vi "Scale Controls.vi"(6 "Initialize group (false)":bool, 7 "rules":string, 8 "error in (no error)":errorcluster, 9 "pane size":T3, 10 "Decorations on Pane":refnum<vi>[](array[refnum]), 11 "Controls on Pane":refnum<vi>[](array[refnum])) -> (0 "error out":errorcluster)   [LabVIEW 2020]
doc: "Simple and schmutzig VI that will scale controls and labeled decorations by delta change of pane size.\nUsage: put in multiline string with rules:\nmy control name a [edge:LRTB]\nmy control name b [edge:LRB]\n...\n\nwhere edge:LRTB defines edges to be sticked to pane. LR - scale horizontaly, R - no scale, move object only, TB - scale vertically, B - just stick object to bottom, no scaling...\nWhen using for decorations, name them first with script 'Set Decoration Label'!"
uses:
  <vilib>/Utility/miscctls.llb/LVRectTypeDef.ctl
  Scale Controls List.ctl
  Scale Controls Record.ctl
  <vilib>/regexp/Match Regular Expression.xnode
panel:
  in  "lists":T1[](array[typedef])
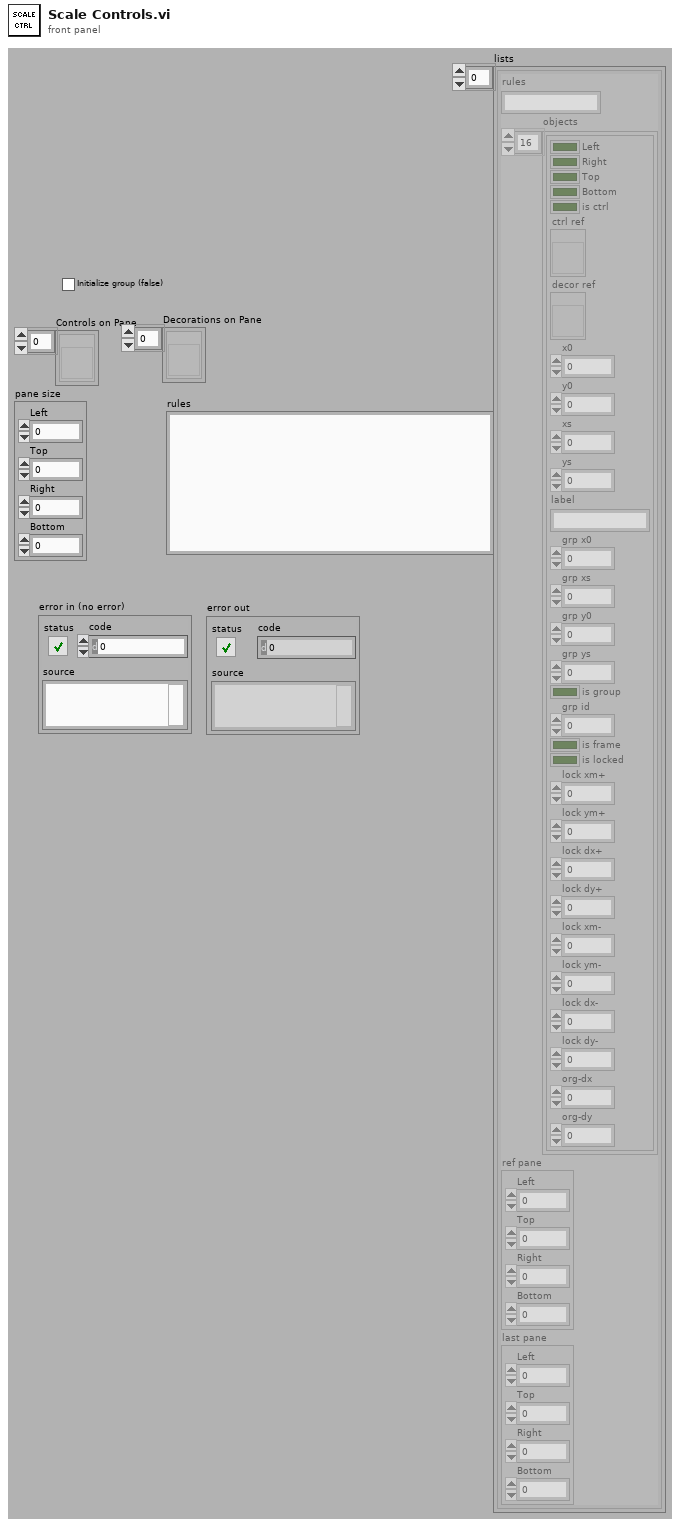
[diagram p1: front panel]
types:
  T1 = typedef "Scale Controls List.ctl" = cluster{"rules":string, "objects":T2[], "ref pane":T3, "last pane":T3}
  T2 = typedef "Scale Controls Record.ctl" = cluster{"Left":bool, "Right":bool, "Top":bool, "Bottom":bool, "is ctrl":bool, "ctrl ref":refnum<vi>, "decor ref":refnum<vi>, "x0":i32, "y0":i32, "xs":i32, "ys":i32, "label":string, "grp x0":i32, "grp xs":i32, "grp y0":i32, "grp ys":i32, "is group":bool, "grp id":i32, "is frame":bool, "is locked":bool, "lock xm+":i32, "lock ym+":i32, "lock dx+":i32, "lock dy+":i32, "lock xm-":i32, "lock ym-":i32, "lock dx-":i32, "lock dy-":i32, "org-dx":i32, "org-dy":i32}
  T3 = typedef "LVRectTypeDef.ctl" = cluster{"Left":i16, "Top":i16, "Right":i16, "Bottom":i16}
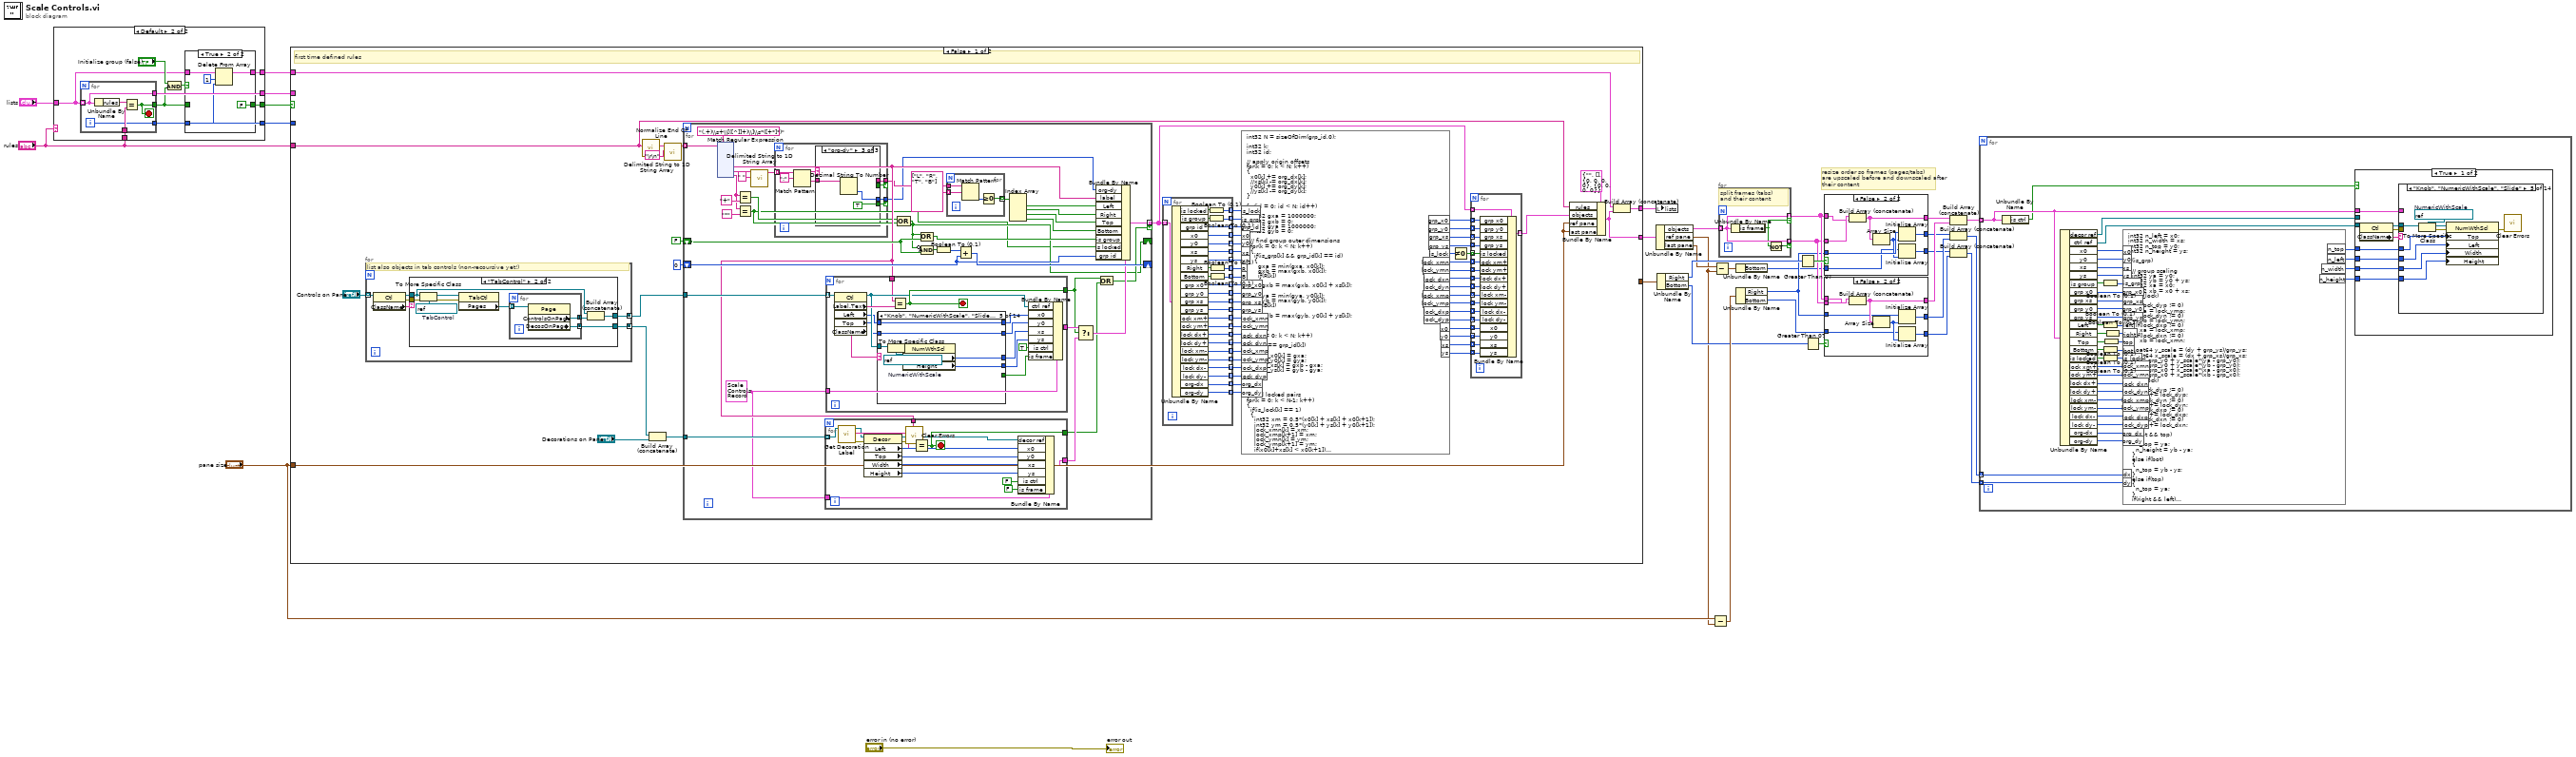
[diagram p0: block diagram]
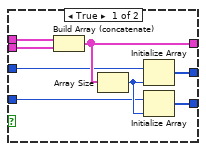
[diagram p2: hidden frame]
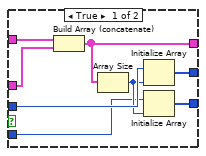
[diagram p3: hidden frame]
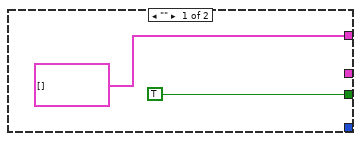
[diagram p4: hidden frame]
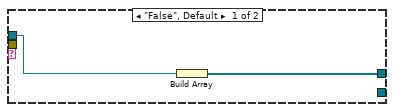
[diagram p6: hidden frame]
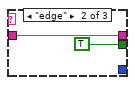
[diagram p8: hidden frame]
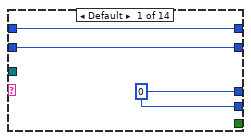
[diagram p9: hidden frame]
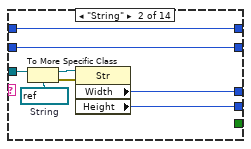
[diagram p10: hidden frame]
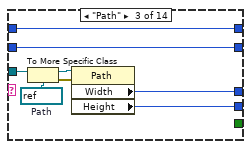
[diagram p11: hidden frame]
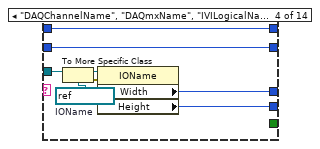
[diagram p12: hidden frame]
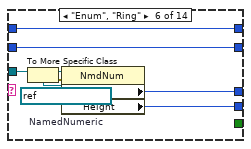
[diagram p13: hidden frame]
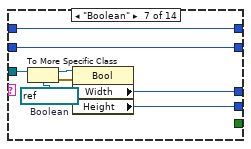
[diagram p14: hidden frame]
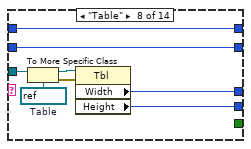
[diagram p15: hidden frame]
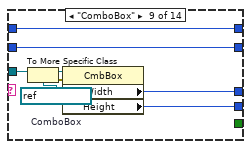
[diagram p16: hidden frame]
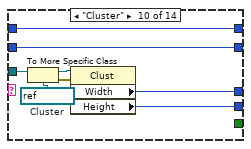
[diagram p17: hidden frame]
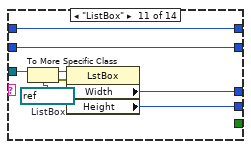
[diagram p18: hidden frame]
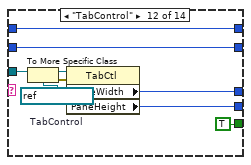
[diagram p19: hidden frame]
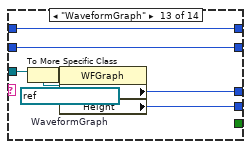
[diagram p20: hidden frame]
diagram:
  # "resize order so frames (pages/tabs)\nare upscaled before and downscaled after\ntheir content"
  n1 = case shown="Default" "rules" {
    tunnel: [TRUE w40] -> w33
    tunnel: [_ w45] -> w31
    tunnel: "rules" -> [_ w44]
    tunnel: [T1[] [] ("lists") w38] -> w29
    tunnel: "lists" -> [_ w39]
    tunnel: [_ w37] -> w9
    frame "" {
    }
    frame Default {
      n2 = for {
        tunnel: w39 -> [w54] mode=indexing
        tunnel: w44 -> [w56]
        tunnel: [w55] -> w41
        tunnel: [w54] -> w45
        tunnel: [w53] -> w37
        i -> [w53]
        stop <- w55 stop-if-true
        n3 = Unbundle By Name(w54) -> ("rules"=w57:string)
        n4 = Equal?(x=w57, y=w56) -> (x = y?=w55:bool)
      }
      n5 = Compound Arithmetic op=AND("Initialize group (false)", w41) -> (w42:bool)
      n6 = case shown="True" w42 {
        tunnel: [w47 FALSE] -> w40
        tunnel: w41 -> [w47 _]
        tunnel: w39 -> [w46 w52]
        tunnel: [w46 w51] -> w38
        tunnel: w37 -> [_ w49]
        frame False {
        }
        frame True {
          n7 = Delete From Array(array=w52, length=1, index=w49) -> (array with subset deleted=w51:T1[])  [unwired: 1 out]
        }
      }
    }
  }
  n8 = case shown="False" w33 {
    tunnel: "rules" -> [w112 _]
    tunnel: w29 -> [w111 w500]
    tunnel: [w110 w499] -> w32
    tunnel: [w109 w498] -> w30
    tunnel: w31 -> [_ w502]
    tunnel: "pane size" -> [w88 w495]
    tunnel: w9 -> [_ w497]
    tunnel: [_ w501] -> w8
    frame False {
      # "first time defined rules"
      n9 = for {
        tunnel: "Controls on Pane" -> [w122] mode=indexing
        tunnel: [w118] -> w61 mode=concatenating
        tunnel: [w117] -> w60 mode=concatenating
        # "list also objects in tab controls (non-recoursive yet!)"
        n10 = property class="Ctl"(reference=w122) -> (reference out=w119:refnum<vi>, error out=w120:errorcluster, "ClassName"=w121:string)  [unwired: 1 in]
        n11 = case shown="\"TabControl\"" w121 {
          tunnel: w120 -> [_ w130]
          tunnel: w119 -> [w124 w127]
          tunnel: [w123 w126] -> w118
          tunnel: [_ w125] -> w117
          frame "False", Default {
            n12 = Build Array(w124) -> (w123:refnum<vi>[])
          }
          frame "TabControl" {
            w131 = refnum<vi> refnum  # TabControl
            n13 = To More Specific Class(target class=w131, reference=w127, error in=w130) -> (specific class reference=w133:refnum<vi>, error out=w132:errorcluster)
            n14 = property class="TabCtl"(reference=w133, error in=w132) -> ("Pages"=w129:refnum<vi>[])  [unwired: 2 out]
            n15 = for {
              tunnel: w129 -> [w136] mode=indexing
              tunnel: [w135] -> w128 mode=concatenating
              tunnel: [w134] -> w125 mode=concatenating
              n16 = property class="Page"(reference=w136) -> ("ControlsOnPage"=w135:refnum<vi>[], "DecosOnPage"=w134:refnum<vi>[])  [unwired: 1 in, 2 out]
            }
            n17 = Build Array (concatenate)(w127, w128) -> (w126:refnum<vi>[])
          }
        }
      }
      n18 = call <vilib>:"Normalize End Of Line.vi"("string in"=w112) -> ("string out"=w114:string)  [unwired: 7 in]
      n19 = Build Array (concatenate)(w60, "Decorations on Pane") -> (w58:refnum<vi>[])
      n20 = call <vilib>:"Delimited String to 1D String Array.vi"("delimiter"="\r\n", "delimited string"=w114) -> ("string array"=w115:string[])  [unwired: 9 in]
      n21 = for {
        tunnel: w115 -> [w219] mode=indexing
        tunnel: [w210] -> w95 mode=indexing if=w195
        tunnel: w61 -> [w211]
        shift-right: [w191] -> _
        shift-left: FALSE -> [w208]
        shift-right: [w205] -> _
        shift-left: 0 -> [w204]
        tunnel: w58 -> [w203]
        w201 = T2 {"Left"=FALSE, "Right"=FALSE, "Top"=FALSE, "Bottom"=FALSE, "is ctrl"=FALSE, "ctrl ref"=refnum, "decor ref"=refnum, "x0"=0, "y0"=0, "xs"=0, "ys"=0, "label"="", "grp x0"=0, "grp xs"=0, "grp y0"=0, "grp ys"=0, "is group"=FALSE, "grp id"=0, "is frame"=FALSE, "is locked"=FALSE, "lock xm+"=0, "lock ym+"=0, "lock dx+"=0, "lock dy+"=0, "lock xm-"=0, "lock ym-"=0, "lock dx-"=0, "lock dy-"=0, "org-dx"=0, "org-dy"=0} ("object")
        n22 = xnode "Match Regular Expression"("input string"=w219, "regular expression"="(.+)\\s+\\[([^]]+)\\]\\s*([+*]*)") -> ("submatch 1"=w202:string, "submatch 2"=w188:string, "submatch 3"=w189:string)  [unwired: 4 in, 5 out]
        n23 = Equal?(x=w189, y="+") -> (x = y?=w192:bool)
        n24 = Equal?(x=w189, y="*") -> (x = y?=w190:bool)
        n25 = call <vilib>:"Delimited String to 1D String Array.vi"("delimiter"=" ", "delimited string"=w188) -> ("string array"=w186:string[])  [unwired: 9 in]
        n26 = for {
          tunnel: w186 -> [w227] mode=indexing
          tunnel: [w223] -> w185 if=w222
          tunnel: [w221] -> w184 if=w220
          n27 = Match Pattern(string=w227, regular expression=":") -> (before substring=w225:string, after substring=w224:string)  [unwired: 1 in, 2 out]
          n28 = case shown="\"org-dy\"" w225 {
            tunnel: [_ w229 _] -> w223
            tunnel: w224 -> [_ w229 w232]
            tunnel: [_ TRUE _] -> w222
            tunnel: [_ _ w231] -> w221
            tunnel: [_ _ TRUE] -> w220
            frame Default {
            }
            frame "edge" {
            }
            frame "org-dy" {
              n29 = Decimal String To Number(string=w232) -> (number=w231:i32)  [unwired: 2 in, 1 out]
            }
          }
        }
        n30 = for {
          tunnel: w203 -> [w237] mode=indexing
          tunnel: w202 -> [w244]
          tunnel: w201 -> [w243]
          tunnel: [w246] -> w199
          tunnel: [w245] -> w196
          stop <- w245 stop-if-true
          n31 = call "Get Decoration Label.vi"("Decor Refnum"=w237) -> ("error out"=w238:errorcluster, "Label"=w239:string, "dup Decor Refnum"=w236:refnum<vi>)  [unwired: 4 in]
          n32 = property class="Decor"(reference=w236, error in=w238) -> (reference out=w235:refnum<vi>, error out=w234:errorcluster, "Left"=w248:i32, "Top"=w242:i32, "Width"=w241:u32, "Height"=w240:u32)
          n33 = call <vilib>:"Clear Errors.vi"("error in (no error)"=w234) -> ()  [unwired: 5 in, 2 out]
          n34 = Equal?(x=w244, y=w239) -> (x = y?=w245:bool)
          n35 = Bundle By Name(cluster=w243, "decor ref"=w235, "x0"=w248, "y0"=w242, "xs"=w241, "ys"=w240, "is ctrl"=FALSE, "is frame"=FALSE) -> (w246:T2)
        }
        n36 = for {
          tunnel: w211 -> [w264] mode=indexing
          tunnel: w202 -> [w257]
          tunnel: w201 -> [w255]
          tunnel: [w261] -> w200
          tunnel: [w260] -> w197
          stop <- w260 stop-if-true
          n37 = property class="Ctl"(reference=w264) -> (reference out=w259:refnum<vi>, "Label.Text"=w263:string, "Left"=w252:i32, "Top"=w250:i32, "ClassName"=w258:string)  [unwired: 1 in, 1 out]
          n38 = case shown="\"Knob\", \"NumericWithScale\", \"Slide\"" w258 {
            tunnel: w259 -> [_ w272 w280 w288 w296 w304 w312 w320 w328 w336 w344 w353 w361 w369]
            tunnel: [w267 w271 w279 w287 w295 w303 w311 w319 w327 w335 w343 w352 w360 w368] -> w256
            tunnel: [w267 w270 w278 w286 w294 w302 w310 w318 w326 w334 w342 w351 w359 w366] -> w254
            tunnel: [_ _ _ _ _ _ _ _ _ _ _ TRUE ("is ctrl") _ _] -> w253
            tunnel: [w265 w269 w277 w285 w293 w301 w309 w317 w325 w333 w341 w349 w358 w367] -> w251
            tunnel: w252 -> [w265 w269 w277 w285 w293 w301 w309 w317 w325 w333 w341 w349 w358 w367]
            tunnel: [w266 w268 w276 w284 w292 w300 w308 w316 w324 w332 w340 w348 w357 w365] -> w249
            tunnel: w250 -> [w266 w268 w276 w284 w292 w300 w308 w316 w324 w332 w340 w348 w357 _]
            frame Default {
              w267 = u32 0 ("Width")
            }
            frame "String" {
              w275 = refnum<vi> refnum  # String
              n39 = To More Specific Class(target class=w275, reference=w272) -> (specific class reference=w273:refnum<vi>, error out=w274:errorcluster)  [unwired: 1 in]
              n40 = property class="Str"(reference=w273, error in=w274) -> ("Width"=w271:u32, "Height"=w270:u32)  [unwired: 2 out]
            }
            frame "Path" {
              w283 = refnum<vi> refnum  # Path
              n41 = To More Specific Class(target class=w283, reference=w280) -> (specific class reference=w281:refnum<vi>, error out=w282:errorcluster)  [unwired: 1 in]
              n42 = property class="Path"(reference=w281, error in=w282) -> ("Width"=w279:u32, "Height"=w278:u32)  [unwired: 2 out]
            }
            frame "DAQChannelName", "DAQmxName", "IVILogicalName", "VISAResourceName" {
              w291 = refnum<vi> refnum  # IOName
              n43 = To More Specific Class(target class=w291, reference=w288) -> (specific class reference=w289:refnum<vi>, error out=w290:errorcluster)  [unwired: 1 in]
              n44 = property class="IOName"(reference=w289, error in=w290) -> ("Width"=w287:u32, "Height"=w286:u32)  [unwired: 2 out]
            }
            frame "Knob", "NumericWithScale", "Slide" {
              w299 = refnum<vi> refnum  # NumericWithScale
              n45 = To More Specific Class(target class=w299, reference=w296) -> (specific class reference=w297:refnum<vi>, error out=w298:errorcluster)  [unwired: 1 in]
              n46 = property class="NumWthScl"(reference=w297, error in=w298) -> ("Width"=w295:u32, "Height"=w294:u32)  [unwired: 2 out]
            }
            frame "Enum", "Ring" {
              w307 = refnum<vi> refnum  # NamedNumeric
              n47 = To More Specific Class(target class=w307, reference=w304) -> (specific class reference=w305:refnum<vi>, error out=w306:errorcluster)  [unwired: 1 in]
              n48 = property class="NmdNum"(reference=w305, error in=w306) -> ("Width"=w303:u32, "Height"=w302:u32)  [unwired: 2 out]
            }
            frame "Boolean" {
              w315 = refnum<vi> refnum  # Boolean
              n49 = To More Specific Class(target class=w315, reference=w312) -> (specific class reference=w313:refnum<vi>, error out=w314:errorcluster)  [unwired: 1 in]
              n50 = property class="Bool"(reference=w313, error in=w314) -> ("Width"=w311:u32, "Height"=w310:u32)  [unwired: 2 out]
            }
            frame "Table" {
              w323 = refnum<vi> refnum  # Table
              n51 = To More Specific Class(target class=w323, reference=w320) -> (specific class reference=w321:refnum<vi>, error out=w322:errorcluster)  [unwired: 1 in]
              n52 = property class="Tbl"(reference=w321, error in=w322) -> ("Width"=w319:u32, "Height"=w318:u32)  [unwired: 2 out]
            }
            frame "ComboBox" {
              w331 = refnum<vi> refnum  # ComboBox
              n53 = To More Specific Class(target class=w331, reference=w328) -> (specific class reference=w329:refnum<vi>, error out=w330:errorcluster)  [unwired: 1 in]
              n54 = property class="CmbBox"(reference=w329, error in=w330) -> ("Width"=w327:u32, "Height"=w326:u32)  [unwired: 2 out]
            }
            frame "Cluster" {
              w339 = refnum<vi> refnum  # Cluster
              n55 = To More Specific Class(target class=w339, reference=w336) -> (specific class reference=w337:refnum<vi>, error out=w338:errorcluster)  [unwired: 1 in]
              n56 = property class="Clust"(reference=w337, error in=w338) -> ("Width"=w335:u32, "Height"=w334:u32)  [unwired: 2 out]
            }
            frame "ListBox" {
              w347 = refnum<vi> refnum  # ListBox
              n57 = To More Specific Class(target class=w347, reference=w344) -> (specific class reference=w345:refnum<vi>, error out=w346:errorcluster)  [unwired: 1 in]
              n58 = property class="LstBox"(reference=w345, error in=w346) -> ("Width"=w343:u32, "Height"=w342:u32)  [unwired: 2 out]
            }
            frame "TabControl" {
              w356 = refnum<vi> refnum  # TabControl
              n59 = To More Specific Class(target class=w356, reference=w353) -> (specific class reference=w354:refnum<vi>, error out=w355:errorcluster)  [unwired: 1 in]
              n60 = property class="TabCtl"(reference=w354, error in=w355) -> ("PaneWidth"=w352:u32, "PaneHeight"=w351:u32)  [unwired: 2 out]
            }
            frame "WaveformGraph" {
              w364 = refnum<vi> refnum  # WaveformGraph
              n61 = To More Specific Class(target class=w364, reference=w361) -> (specific class reference=w362:refnum<vi>, error out=w363:errorcluster)  [unwired: 1 in]
              n62 = property class="WFGraph"(reference=w362, error in=w363) -> ("Width"=w360:u32, "Height"=w359:u32)  [unwired: 2 out]
            }
            frame "XYGraph" {
              w372 = refnum<vi> refnum  # XYGraph
              n63 = To More Specific Class(target class=w372, reference=w369) -> (specific class reference=w370:refnum<vi>, error out=w371:errorcluster)  [unwired: 1 in]
              n64 = property class="XYGraph"(reference=w370, error in=w371) -> ("Width"=w368:u32, "Height"=w366:u32, "Top"=w365:i32)  [unwired: 2 out]
            }
          }
          n65 = Equal?(x=w257, y=w263) -> (x = y?=w260:bool)
          n66 = Bundle By Name(cluster=w255, "ctrl ref"=w259, "x0"=w251, "y0"=w249, "xs"=w256, "ys"=w254, "is ctrl"=TRUE, "is frame"=w253) -> (w261:T2)
        }
        n67 = Compound Arithmetic op=OR(w192, w190) -> (w191:bool)
        n68 = Compound Arithmetic op=OR(w191, w208) -> (w193:bool)
        n69 = Compound Arithmetic op=AND(invert w191, w208) -> (w207:bool)
        n70 = Boolean To (0,1)(Boolean=w207) -> (0, 1=w206:i16)
        n71 = for {
          tunnel: w185 -> [w376]
          tunnel: string[] ["L", "R", "T", "B"] -> [w375] mode=indexing
          tunnel: [w373] -> w216 mode=indexing
          n72 = Match Pattern(string=w376, regular expression=w375) -> (offset past match=w374:i32)  [unwired: 1 in, 3 out]
          n73 = Greater Or Equal To 0?(x=w374) -> (x >= 0?=w373:bool)
        }
        n74 = Add(x=w206, y=w204) -> (x+y=w205:i32)
        n75 = Index Array(array=w216) -> (element #1=w215:bool, element #2=w214:bool, element #3=w213:bool, element #4=w212:bool)  [unwired: 4 in]
        n76 = Select(t=w200, s=w197, f=w199) -> (s? t:f=w198:T2)
        n77 = Bundle By Name(cluster=w198, "org-dy"=w184, "label"=w202, "Left"=w215, "Right"=w214, "Top"=w213, "Bottom"=w212, "is group"=w193, "is locked"=w190, "grp id"=w204) -> (w210:T2)
        n78 = Compound Arithmetic op=OR(w197, w196) -> (w195:bool)
      }
      n79 = for {
        tunnel: w95 -> [w183] mode=indexing
        tunnel: [w181] -> w106 mode=indexing
        tunnel: [w180] -> w89 mode=indexing
        tunnel: [w179] -> w105 mode=indexing
        tunnel: [w178] -> w104 mode=indexing
        tunnel: [w177] -> w103 mode=indexing
        tunnel: [w176] -> w102 mode=indexing
        tunnel: [w174] -> w101 mode=indexing
        tunnel: [w172] -> w100 mode=indexing
        tunnel: [w171] -> w99 mode=indexing
        tunnel: [w170] -> w98 mode=indexing
        tunnel: [w169] -> w97 mode=indexing
        tunnel: [w168] -> w96 mode=indexing
        tunnel: [w166] -> w87 mode=indexing
        tunnel: [w165] -> w80 mode=indexing
        tunnel: [w164] -> w79 mode=indexing
        tunnel: [w163] -> w78 mode=indexing
        tunnel: [w162] -> w77 mode=indexing
        tunnel: [w161] -> w76 mode=indexing
        tunnel: [w160] -> w75 mode=indexing
        tunnel: [w159] -> w74 mode=indexing
        tunnel: [w158] -> w73 mode=indexing
        tunnel: [w157] -> w68 mode=indexing
        tunnel: [w156] -> w67 mode=indexing
        n80 = Unbundle By Name(w183) -> ("is locked"=w167:bool, "is group"=w182:bool, "grp id"=w181:i32, "x0"=w179:i32, "y0"=w178:i32, "xs"=w177:i32, "ys"=w176:i32, "Right"=w175:bool, "Bottom"=w173:bool, "grp x0"=w171:i32, "grp y0"=w170:i32, "grp xs"=w169:i32, "grp ys"=w168:i32, "lock xm+"=w165:i32, "lock ym+"=w164:i32, "lock dx+"=w163:i32, "lock dy+"=w162:i32, "lock xm-"=w161:i32, "lock ym-"=w160:i32, "lock dx-"=w159:i32, "lock dy-"=w158:i32, "org-dx"=w157:i32, "org-dy"=w156:i32)
        n81 = Boolean To (0,1)(Boolean=w167) -> (0, 1=w166:i16)
        n82 = Boolean To (0,1)(Boolean=w182) -> (0, 1=w180:i16)
        n83 = Boolean To (0,1)(Boolean=w175) -> (0, 1=w174:i16)
        n84 = Boolean To (0,1)(Boolean=w173) -> (0, 1=w172:i16)
      }
      n85 = formula code="int32 N = sizeOfDim(grp_id,0);\n\nint32 k;\nint32 id;\n\n// apply origin offsets\nfor(k = 0; k < N; k++)\n{\n  x0[k] += org_dx[k];\n  //xs[k] -= org_dx[k];\n  y0[k] += org_dy[k];\n  //ys[k] -= org_dy[k];\n}\n\nfor(id = 0; id < N; id++)\n{\n  int32 gxa = 1000000;\n  int32 gxb = 0;\n  int32 gya = 1000000;\n  int32 gyb = 0;\n\n  // find group outer dimensions\n  for(k = 0; k < N; k++)\n  {\n    if(is_grp[k] && grp_id[k] == id)\n    {\n      gxa = min(gxa, x0[k]);\n      gxb = max(gxb, x0[k]);\n      if(R[k])\n      {\n        gxb = max(gxb, x0[k] + xs[k]);\n      }\n      gya = min(gya, y0[k]);\n      gyb = max(gyb, y0[k]);\n      if(B[k])\n      {\n        gyb = max(gyb, y0[k] + ys[k]);\n      }\n    }\n  }\n  for(k = 0; k < N; k++)\n  {\n    if(id == grp_id[k])\n    {\n      grp_x0[k] = gxa;\n      grp_y0[k] = gya;\n      grp_xs[k] = gxb - gxa;\n      grp_ys[k] = gyb - gya;\n    }\n  }\n}\n\n// find locked pairs\nfor(k = 0; k < N-1; k++)\n{\n  if(is_lock[k] == 1)\n  {\n    int32 xm = 0.5*(x0[k] + xs[k] + x0[k+1]);\n    int32 ym = 0.5*(y0[k] + ys[k] + y0[k+1]);\n    lock_xmn[k] = xm;\n    lock_xmp[k+1] = xm;\n    lock_ymn[k] = ym;\n    lock_ymp[k+1] = ym;\n    if(x0[k]+xs[k] < x0[k+1])\n    {\n      lock_dxn[k] = (x0[k] + xs[k]) - xm;\n      lock_dxp[k+1] = (x0[k+1]) - xm;\n    }\n    else\n    {\n      lock_dxn[k] = 0;\n      lock_dxp[k+1] = 0;\n    }\n    if(y0[k]+ys[k] < y0[k+1])\n    {\n      lock_dyn[k] = (y0[k] + ys[k]) - ym;\n      lock_dyp[k+1] = (y0[k+1]) - ym;\n    }\n    else\n    {\n      lock_dyn[k] = 0;\n      lock_dyp[k+1] = 0;\n    }\n    if(!is_lock[k+1])\n      is_lock[k+1] = 2;\n  }\n}"("is_grp"=w89, "grp_id"=w106, "x0"=w105, "y0"=w104, "xs"=w103, "ys"=w102, "R"=w101, "B"=w100, "grp_x0"=w99, "grp_y0"=w98, "grp_xs"=w97, "grp_ys"=w96, "is_lock"=w87, "lock_xmn"=w80, "lock_ymn"=w79, "lock_dxn"=w78, "lock_dyn"=w77, "lock_xmp"=w76, "lock_ymp"=w75, "lock_dxp"=w74, "lock_dyp"=w73, "org_dx"=w68, "org_dy"=w67) -> ("grp_x0"=w94:i32[], "grp_y0"=w93:i32[], "grp_xs"=w92:i32[], "grp_ys"=w91:i32[], "is_lock"=w86:i16[], "lock_xmn"=w84:i32[], "lock_ymn"=w83:i32[], "lock_dxn"=w82:i32[], "lock_dyn"=w81:i32[], "lock_xmp"=w72:i32[], "lock_ymp"=w71:i32[], "lock_dxp"=w70:i32[], "lock_dyp"=w69:i32[], "x0"=w66:i32[], "y0"=w65:i32[], "xs"=w64:i32[], "ys"=w63:i32[])
      n86 = Not Equal To 0?(x=w86) -> (x != 0?=w85:bool[])
      n87 = for {
        tunnel: w95 -> [w155] mode=indexing
        tunnel: w94 -> [w154] mode=indexing
        tunnel: w93 -> [w153] mode=indexing
        tunnel: w92 -> [w152] mode=indexing
        tunnel: w91 -> [w151] mode=indexing
        tunnel: [w150] -> w90 mode=indexing
        tunnel: w85 -> [w149] mode=indexing
        tunnel: w84 -> [w148] mode=indexing
        tunnel: w83 -> [w147] mode=indexing
        tunnel: w82 -> [w146] mode=indexing
        tunnel: w81 -> [w145] mode=indexing
        tunnel: w72 -> [w144] mode=indexing
        tunnel: w71 -> [w143] mode=indexing
        tunnel: w70 -> [w142] mode=indexing
        tunnel: w69 -> [w141] mode=indexing
        tunnel: w66 -> [w140] mode=indexing
        tunnel: w65 -> [w139] mode=indexing
        tunnel: w64 -> [w138] mode=indexing
        tunnel: w63 -> [w137] mode=indexing
        n88 = Bundle By Name(cluster=w155, "grp x0"=w154, "grp y0"=w153, "grp xs"=w152, "grp ys"=w151, "is locked"=w149, "lock xm+"=w148, "lock ym+"=w147, "lock dx+"=w146, "lock dy+"=w145, "lock xm-"=w144, "lock ym-"=w143, "lock dx-"=w142, "lock dy-"=w141, "x0"=w140, "y0"=w139, "xs"=w138, "ys"=w137) -> (w150:T2)
      }
      n89 = Bundle By Name(cluster=T1 {"rules"="", "objects"=[], "ref pane"={"Left"=0, "Top"=0, "Right"=0, "Bottom"=0}, "last pane"={"Left"=0, "Top"=0, "Right"=0, "Bottom"=0}} ("obj list"), "rules"=w112, "objects"=w90, "ref pane"=w88, "last pane"=w88) -> (w109:T1)
      n90 = Build Array (concatenate)(w111, w109) -> (w110:T1[])
    }
    frame True {
      # "old rules found"
      n91 = Unbundle By Name(w502) -> ("last pane"=w496:T3)
      n92 = Subtract(x=w495, y=w496) -> (x-y=w501:T3)
      n93 = Bundle By Name(cluster=w502, "last pane"=w495) -> (w498:T1)
      n94 = Replace Array Subset(array=w500, new element=w498, index=w497) -> (w499:T1[])
    }
  }
  n95 = local write "lists"(w32) -> ()
  n96 = Unbundle By Name(w30) -> ("objects"=w25:T2[], "ref pane"=w2:T3, "last pane"=w3:T3)
  n97 = Unbundle By Name(w8) -> ("Right"=w7:i16, "Bottom"=w6:i16)
  n98 = Subtract(x="pane size", y=w2) -> (x-y=w23:T3)
  n99 = Subtract(x=w3, y=w2) -> (x-y=w1:T3)
  n100 = for {
    tunnel: w25 -> [w505] mode=indexing
    tunnel: [w505] -> w20 mode=indexing if=w503
    tunnel: [w505] -> w19 mode=indexing if=w504
    # "split frames (tabs)\nand their content"
    n101 = Unbundle By Name(w505) -> ("is frame"=w503:bool)
    n102 = Not(x=w503) -> (.not. x?=w504:bool)
  }
  n103 = Unbundle By Name(w1) -> ("Bottom"=w4:i16)
  n104 = Unbundle By Name(w23) -> ("Right"=w5:i16, "Bottom"=w21:i16)
  n105 = Greater Than 0?(x=w7) -> (x > 0?=w24:bool)
  n106 = Greater Than 0?(x=w6) -> (x > 0?=w22:bool)
  n107 = case shown="False" w24 {
    tunnel: w20 -> [w513 w515]
    tunnel: w19 -> [w512 w516]
    tunnel: [w511 w521] -> w18
    tunnel: [w510 w520] -> w16
    tunnel: w5 -> [w509 w519]
    tunnel: [w507 w517] -> w14
    tunnel: w4 -> [w506 w514]
    frame True {
      n108 = Build Array (concatenate)(w513, w512) -> (w511:T2[])
      n109 = Array Size(array=w511) -> (size(s)=w508:i32)
      n110 = Initialize Array(w509, w508) -> (w510:i16[])
      n111 = Initialize Array(w506, w508) -> (w507:i16[])
    }
    frame False {
      n112 = Build Array (concatenate)(w516, w515) -> (w521:T2[])
      n113 = Array Size(array=w521) -> (size(s)=w518:i32)
      n114 = Initialize Array(w519, w518) -> (w520:i16[])
      n115 = Initialize Array(w514, w518) -> (w517:i16[])
    }
  }
  n116 = case shown="False" w22 {
    tunnel: w20 -> [w529 w532]
    tunnel: w19 -> [w528 w533]
    tunnel: [w527 w537] -> w17
    tunnel: [w526 w536] -> w15
    tunnel: w21 -> [w523 w531]
    tunnel: [w524 w534] -> w13
    tunnel: w5 -> [w522 w530]
    frame True {
      n117 = Build Array (concatenate)(w529, w528) -> (w527:T2[])
      n118 = Array Size(array=w527) -> (size(s)=w525:i32)
      n119 = Initialize Array(w522, w525) -> (w526:i16[])
      n120 = Initialize Array(w523, w525) -> (w524:i16[])
    }
    frame False {
      n121 = Build Array (concatenate)(w533, w532) -> (w537:T2[])
      n122 = Array Size(array=w537) -> (size(s)=w535:i32)
      n123 = Initialize Array(w530, w535) -> (w536:i16[])
      n124 = Initialize Array(w531, w535) -> (w534:i16[])
    }
  }
  n125 = Build Array (concatenate)(w18, w17) -> (w12:T2[])
  n126 = Build Array (concatenate)(w16, w15) -> (w11:i16[])
  n127 = Build Array (concatenate)(w14, w13) -> (w10:i16[])
  n128 = for {
    tunnel: w12 -> [w577] mode=indexing
    tunnel: w11 -> [w551] mode=indexing
    tunnel: w10 -> [w550] mode=indexing
    n129 = Unbundle By Name(w577) -> ("is ctrl"=w553:bool)
    n130 = Unbundle By Name(w577) -> ("decor ref"=w552:refnum<vi>, "ctrl ref"=w576:refnum<vi>, "x0"=w575:i32, "y0"=w574:i32, "xs"=w573:i32, "ys"=w572:i32, "is group"=w571:bool, "grp x0"=w569:i32, "grp xs"=w567:i32, "grp y0"=w568:i32, "grp ys"=w566:i32, "Left"=w565:bool, "Right"=w563:bool, "Top"=w561:bool, "Bottom"=w559:bool, "is locked"=w549:bool, "lock xm+"=w547:i32, "lock ym+"=w546:i32, "lock dx+"=w545:i32, "lock dy+"=w544:i32, "lock xm-"=w543:i32, "lock ym-"=w542:i32, "lock dx-"=w541:i32, "lock dy-"=w540:i32, "org-dx"=w539:i32, "org-dy"=w538:i32)
    n131 = Boolean To (0,1)(Boolean=w565) -> (0, 1=w564:i16)
    n132 = Boolean To (0,1)(Boolean=w571) -> (0, 1=w570:i16)
    n133 = Boolean To (0,1)(Boolean=w559) -> (0, 1=w558:i16)
    n134 = Boolean To (0,1)(Boolean=w549) -> (0, 1=w548:i16)
    n135 = Boolean To (0,1)(Boolean=w561) -> (0, 1=w560:i16)
    n136 = Boolean To (0,1)(Boolean=w563) -> (0, 1=w562:i16)
    n137 = formula code="int32 n_left = x0;\nint32 n_width = xs;\nint32 n_top = y0;\nint32 n_height = ys;\n\nif(is_grp)\n{\n  // group scaling\n  int32 ya = y0;\n  int32 yb = y0 + ys;\n  int32 xa = x0;\n  int32 xb = x0 + xs;\n  if(is_lock)\n  {\n    if(lock_dyp != 0)\n      ya = lock_ymp;\n    if(lock_dyn != 0)\n      yb = lock_ymn;\n    if(lock_dxp != 0)\n      xa = lock_xmp;\n    if(lock_dxn != 0)\n      xb = lock_xmn;\n  }\n  float64 y_scale = (dy + grp_ys)/grp_ys;\n  float64 x_scale = (dx + grp_xs)/grp_xs;\n  ya = grp_y0 + y_scale*(ya - grp_y0);\n  yb = grp_y0 + y_scale*(yb - grp_y0);\n  xa = grp_x0 + x_scale*(xa - grp_x0);\n  xb = grp_x0 + x_scale*(xb - grp_x0);\n  if(is_lock)\n  {\n    if(lock_dyp != 0)\n      ya += lock_dyp;\n    if(lock_dyn != 0)\n      yb += lock_dyn;\n    if(lock_dxp != 0)\n      xa += lock_dxp;\n    if(lock_dxn != 0)\n      xb += lock_dxn;\n  }\n  if(bot && top)\n  {\n    n_top = ya;\n    n_height = yb - ya;\n  }\n  else if(bot)\n  {\n    n_top = yb - ys;\n  }\n  else if(top)\n  {\n    n_top = ya;\n  }\n  if(right && left)\n  {\n    n_left = xa;\n    n_width = xb - xa;\n  }\n  else if(right)\n  {\n    n_left = xb - xs;\n  }\n  else if(left)\n  {\n    n_left = xa;\n  }\n}\nelse\n{\n  if(bot && top)\n    n_height = ys + dy;\n  if(bot && !top)\n    n_top = y0 + dy;\n  if(right && left)\n    n_width = xs + dx;\n  if(right && !left)\n    n_left = x0 + dx;\n}\n\nn_left -= org_dx;\n//n_width += org_dx;\nn_top -= org_dy;\n//n_height += org_dy;"("x0"=w575, "y0"=w574, "xs"=w573, "ys"=w572, "is_grp"=w570, "grp_x0"=w569, "grp_y0"=w568, "grp_xs"=w567, "grp_ys"=w566, "left"=w564, "right"=w562, "top"=w560, "bot"=w558, "dx"=w551, "dy"=w550, "is_lock"=w548, "lock_xmn"=w547, "lock_ymn"=w546, "lock_dxn"=w545, "lock_dyn"=w544, "lock_xmp"=w543, "lock_ymp"=w542, "lock_dxp"=w541, "lock_dyp"=w540, "org_dx"=w539, "org_dy"=w538) -> ("n_top"=w557:i32, "n_left"=w556:i32, "n_width"=w555:i32, "n_height"=w554:i32)
    n138 = case shown="True" w553 {
      tunnel: w577 -> [w586 _]
      tunnel: w576 -> [w583 _]
      tunnel: w557 -> [w581 w707]
      tunnel: w556 -> [w580 w706]
      tunnel: w555 -> [w579 w705]
      tunnel: w554 -> [w578 w704]
      tunnel: w552 -> [_ w702]
      frame True {
        n139 = property class="Ctl"(reference=w583) -> (reference out=w585:refnum<vi>, error out=w582:errorcluster, "ClassName"=w584:string)  [unwired: 1 in]
        n140 = case shown="\"Knob\", \"NumericWithScale\", \"Slide\"" w584 {
          tunnel: w585 -> [_ w595 w604 w613 w622 w631 w640 w649 w658 w667 w676 w683 w692 w701]
          tunnel: w586 -> [_ _ _ _ _ _ _ _ _ _ _ _ _ _]
          tunnel: w582 -> [_ _ _ _ _ _ _ _ _ _ _ _ _ _]
          tunnel: w581 -> [_ w591 w600 w609 w618 w627 w636 w645 w654 w663 w672 w679 w684 w697]
          tunnel: w580 -> [_ w590 w599 w608 w617 w626 w635 w644 w653 w662 w671 w678 w688 w696]
          tunnel: w579 -> [_ w589 w598 w607 w616 w625 w634 w643 w652 w661 w670 _ w687 w695]
          tunnel: w578 -> [_ w588 w597 w606 w615 w624 w633 w642 w651 w660 w669 _ w685 w694]
          frame Default {
          }
          frame "String" {
            w593 = refnum<vi> refnum  # String
            n141 = To More Specific Class(target class=w593, reference=w595) -> (specific class reference=w594:refnum<vi>, error out=w592:errorcluster)  [unwired: 1 in]
            n142 = property class="Str"(reference=w594, error in=w592, "Top"=w591, "Left"=w590, "Width"=w589, "Height"=w588) -> (error out=w587:errorcluster)  [unwired: 1 out]
            n143 = call <vilib>:"Clear Errors.vi"("error in (no error)"=w587) -> ()  [unwired: 5 in, 2 out]
          }
          frame "Path" {
            w602 = refnum<vi> refnum  # Path
            n144 = To More Specific Class(target class=w602, reference=w604) -> (specific class reference=w603:refnum<vi>, error out=w601:errorcluster)  [unwired: 1 in]
            n145 = property class="Path"(reference=w603, error in=w601, "Top"=w600, "Left"=w599, "Width"=w598, "Height"=w597) -> (error out=w596:errorcluster)  [unwired: 1 out]
            n146 = call <vilib>:"Clear Errors.vi"("error in (no error)"=w596) -> ()  [unwired: 5 in, 2 out]
          }
          frame "DAQChannelName", "DAQmxName", "IVILogicalName", "VISAResourceName" {
            w611 = refnum<vi> refnum  # IOName
            n147 = To More Specific Class(target class=w611, reference=w613) -> (specific class reference=w612:refnum<vi>, error out=w610:errorcluster)  [unwired: 1 in]
            n148 = property class="IOName"(reference=w612, error in=w610, "Top"=w609, "Left"=w608, "Width"=w607, "Height"=w606) -> (error out=w605:errorcluster)  [unwired: 1 out]
            n149 = call <vilib>:"Clear Errors.vi"("error in (no error)"=w605) -> ()  [unwired: 5 in, 2 out]
          }
          frame "Knob", "NumericWithScale", "Slide" {
            w620 = refnum<vi> refnum  # NumericWithScale
            n150 = To More Specific Class(target class=w620, reference=w622) -> (specific class reference=w621:refnum<vi>, error out=w619:errorcluster)  [unwired: 1 in]
            n151 = property class="NumWthScl"(reference=w621, error in=w619, "Top"=w618, "Left"=w617, "Width"=w616, "Height"=w615) -> (error out=w614:errorcluster)  [unwired: 1 out]
            n152 = call <vilib>:"Clear Errors.vi"("error in (no error)"=w614) -> ()  [unwired: 5 in, 2 out]
          }
          frame "Enum", "Ring" {
            w629 = refnum<vi> refnum  # NamedNumeric
            n153 = To More Specific Class(target class=w629, reference=w631) -> (specific class reference=w630:refnum<vi>, error out=w628:errorcluster)  [unwired: 1 in]
            n154 = property class="NmdNum"(reference=w630, error in=w628, "Top"=w627, "Left"=w626, "Width"=w625, "Height"=w624) -> (error out=w623:errorcluster)  [unwired: 1 out]
            n155 = call <vilib>:"Clear Errors.vi"("error in (no error)"=w623) -> ()  [unwired: 5 in, 2 out]
          }
          frame "Boolean" {
            w638 = refnum<vi> refnum  # Boolean
            n156 = To More Specific Class(target class=w638, reference=w640) -> (specific class reference=w639:refnum<vi>, error out=w637:errorcluster)  [unwired: 1 in]
            n157 = property class="Bool"(reference=w639, error in=w637, "Top"=w636, "Left"=w635, "Width"=w634, "Height"=w633) -> (error out=w632:errorcluster)  [unwired: 1 out]
            n158 = call <vilib>:"Clear Errors.vi"("error in (no error)"=w632) -> ()  [unwired: 5 in, 2 out]
          }
          frame "Table" {
            w647 = refnum<vi> refnum  # Table
            n159 = To More Specific Class(target class=w647, reference=w649) -> (specific class reference=w648:refnum<vi>, error out=w646:errorcluster)  [unwired: 1 in]
            n160 = property class="Tbl"(reference=w648, error in=w646, "Top"=w645, "Left"=w644, "Width"=w643, "Height"=w642) -> (error out=w641:errorcluster)  [unwired: 1 out]
            n161 = call <vilib>:"Clear Errors.vi"("error in (no error)"=w641) -> ()  [unwired: 5 in, 2 out]
          }
          frame "TabControl" {
            w656 = refnum<vi> refnum  # TabControl
            n162 = To More Specific Class(target class=w656, reference=w658) -> (specific class reference=w657:refnum<vi>, error out=w655:errorcluster)  [unwired: 1 in]
            n163 = property class="TabCtl"(reference=w657, error in=w655, "Top"=w654, "Left"=w653, "PaneWidth"=w652, "PaneHeight"=w651) -> (error out=w650:errorcluster)  [unwired: 1 out]
            n164 = call <vilib>:"Clear Errors.vi"("error in (no error)"=w650) -> ()  [unwired: 5 in, 2 out]
          }
          frame "ComboBox" {
            w665 = refnum<vi> refnum  # ComboBox
            n165 = To More Specific Class(target class=w665, reference=w667) -> (specific class reference=w666:refnum<vi>, error out=w664:errorcluster)  [unwired: 1 in]
            n166 = property class="CmbBox"(reference=w666, error in=w664, "Top"=w663, "Left"=w662, "Width"=w661, "Height"=w660) -> (error out=w659:errorcluster)  [unwired: 1 out]
            n167 = call <vilib>:"Clear Errors.vi"("error in (no error)"=w659) -> ()  [unwired: 5 in, 2 out]
          }
          frame "ListBox" {
            w674 = refnum<vi> refnum  # ListBox
            n168 = To More Specific Class(target class=w674, reference=w676) -> (specific class reference=w675:refnum<vi>, error out=w673:errorcluster)  [unwired: 1 in]
            n169 = property class="LstBox"(reference=w675, error in=w673, "Top"=w672, "Left"=w671, "Width"=w670, "Height"=w669) -> (error out=w668:errorcluster)  [unwired: 1 out]
            n170 = call <vilib>:"Clear Errors.vi"("error in (no error)"=w668) -> ()  [unwired: 5 in, 2 out]
          }
          frame "Cluster" {
            w681 = refnum<vi> refnum  # Cluster
            n171 = To More Specific Class(target class=w681, reference=w683) -> (specific class reference=w682:refnum<vi>, error out=w680:errorcluster)  [unwired: 1 in]
            n172 = property class="Clust"(reference=w682, error in=w680, "Top"=w679, "Left"=w678) -> (error out=w677:errorcluster)  [unwired: 1 out]
            n173 = call <vilib>:"Clear Errors.vi"("error in (no error)"=w677) -> ()  [unwired: 5 in, 2 out]
          }
          frame "XYGraph" {
            w690 = refnum<vi> refnum  # XYGraph
            n174 = To More Specific Class(target class=w690, reference=w692) -> (specific class reference=w691:refnum<vi>, error out=w689:errorcluster)  [unwired: 1 in]
            n175 = property class="XYGraph"(reference=w691, error in=w689, "Top"=w684, "Left"=w688, "Width"=w687, "Height"=w685) -> (error out=w686:errorcluster)  [unwired: 1 out]
            n176 = call <vilib>:"Clear Errors.vi"("error in (no error)"=w686) -> ()  [unwired: 5 in, 2 out]
          }
          frame "WaveformGraph" {
            w699 = refnum<vi> refnum  # WaveformGraph
            n177 = To More Specific Class(target class=w699, reference=w701) -> (specific class reference=w700:refnum<vi>, error out=w698:errorcluster)  [unwired: 1 in]
            n178 = property class="WFGraph"(reference=w700, error in=w698, "Top"=w697, "Left"=w696, "Width"=w695, "Height"=w694) -> (error out=w693:errorcluster)  [unwired: 1 out]
            n179 = call <vilib>:"Clear Errors.vi"("error in (no error)"=w693) -> ()  [unwired: 5 in, 2 out]
          }
        }
      }
      frame False {
        n180 = property class="Decor"(reference=w702, "Top"=w707, "Left"=w706, "Width"=w705, "Height"=w704) -> (error out=w703:errorcluster)  [unwired: 1 in, 1 out]
        n181 = call <vilib>:"Clear Errors.vi"("error in (no error)"=w703) -> ()  [unwired: 5 in, 2 out]
      }
    }
  }
  "error out" <- "error in (no error)"
